vi "SLL DE File Looging Command LV2Global.vi"(6 "Option":T2=enum."Get Event Refnum", 8 "Error in (no error)":errorcluster, 11 "File Logging Option":T1=enum."Stop Logging") -> (0 "Error out":errorcluster, 3 "Event Registration Refnum":refnum<event-registration>)   [LabVIEW 2009]
uses:
  DAQ Engine/Controls/SLL DE DO Command LV2Global Options.ctl
  Controls/SLL DE File Logging Command List.ctl
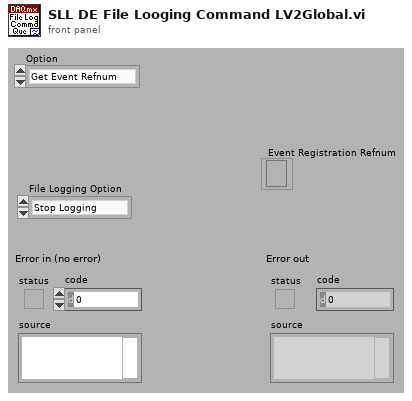
[diagram p1: front panel]
types:
  T1 = typedef "SLL DE File Logging Command List.ctl" = enum16{"Start Logging", "Stop Logging"}
  T2 = typedef "SLL DE DO Command LV2Global Options.ctl" = enum16{"Init/Register Events", "Get Event Refnum", "Fire Event", "Destroy Event"}
  T3 = cluster{"Event Registration Refnum":refnum<event-registration>, "File Logging User Event":refnum<user-event>}
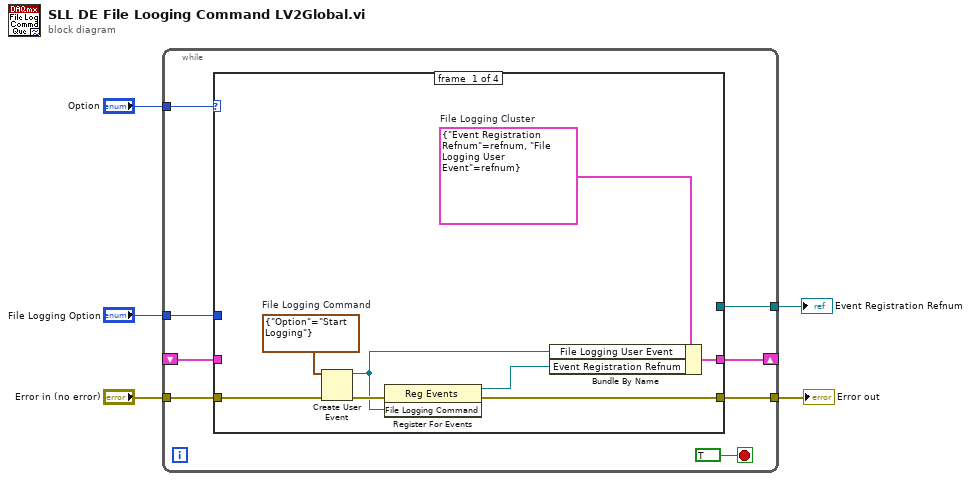
[diagram p0: block diagram]
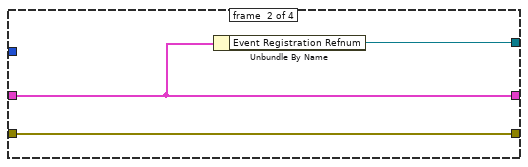
[diagram p2: hidden frame]
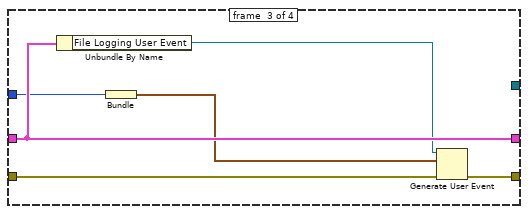
[diagram p3: hidden frame]
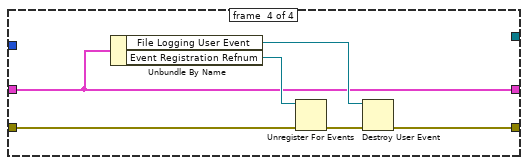
[diagram p4: hidden frame]
diagram:
  n1 = while {
    tunnel: "Option" -> [w12]
    shift-right: [w11] -> _
    shift-left: _ -> [w10]
    tunnel: "File Logging Option" -> [w9]
    tunnel: [w8] -> w3
    tunnel: "Error in (no error)" -> [w7]
    tunnel: [w6] -> w1
    stop <- TRUE stop-if-true
    n2 = case shown="\"Init/Register Events\"" w12 {
      tunnel: [w18 w23 w30 w31] -> w11
      tunnel: w10 -> [_ w23 w30 w31]
      tunnel: w9 -> [_ _ w26 _]
      tunnel: [w17 w24 w27 w32] -> w8
      tunnel: w7 -> [w16 w24 w28 w33]
      tunnel: [_ w22 _ _] -> w6
      frame #0 {
        w21 = T3 {"Event Registration Refnum"=refnum, "File Logging User Event"=refnum}  # File Logging Cluster
        w19 = cluster{"Option":T1} {"Option"=enum."Start Logging"}  # File Logging Command
        n3 = Create User Event(user event datatype=w19, error in=w16) -> (user event=w15:refnum<user-event>, error out=w20:errorcluster)
        n4 = register-events(error in=w20, w15) -> (reference out=w14:refnum<event-registration>, error out=w17:errorcluster)  [unwired: 1 in]
        n5 = Bundle By Name(cluster=w21, "File Logging User Event"=w15, "Event Registration Refnum"=w14) -> (w18:T3)
      }
      frame #1 {
        n6 = Unbundle By Name(w23) -> ("Event Registration Refnum"=w22:refnum<event-registration>)
      }
      frame #2 {
        n7 = Unbundle By Name(w30) -> ("File Logging User Event"=w29:refnum<user-event>)
        n8 = Bundle("File Logging Option"=w26) -> (w25:cluster{"File Logging Option":T1})  [unwired: 1 in]
        n9 = Generate User Event(user event=w29, event data cluster=w25, error in=w28) -> (error out=w27:errorcluster)  [unwired: 1 out]
      }
      frame #3 {
        n10 = Unbundle By Name(w31) -> ("File Logging User Event"=w36:refnum<user-event>, "Event Registration Refnum"=w34:refnum<event-registration>)
        n11 = Unregister For Events(event registration refnum=w34, error in=w33) -> (error out=w35:errorcluster)
        n12 = Destroy User Event(user event=w36, error in=w35) -> (error out=w32:errorcluster)
      }
    }
  }
  "Error out" <- w3
  "Event Registration Refnum" <- w1
